vi "motion_ui.vi"() -> ()   [LabVIEW 2012]
uses:
  <vilib>/Platform/TimedLoop/XDataNode/timing_clust.ctl
  <vilib>/Platform/TimedLoop/XDataNode/nitl_modes.ctl
  <vilib>/Platform/TimedLoop/XDataNode/wakeup.ctl
  <vilib>/Platform/TimedLoop/XDataNode/XDataNode.xnode
  <vilib>/Platform/TimedLoop/XDataNode/XDNodeRunTimeDep.lvlib
panel:
  in  "Axis offsets":dbl[](array[numeric])
  in  "Home position":dbl[](array[numeric])
  in  "End transform":dbl[](array[numeric])
  out "Pose":dbl[](array[numeric]) format="%#.4f"
  out "Axis positions":dbl[](array[numeric]) format="%#.4f"
  in  "Continuous":bool
  in  "Go button":bool
  in  "Axis positions ctl":dbl[](array[numeric])=[0.0]
  in  "Position mode":enum16{"Absolute axis", "Relative axis", "Pose"}(ring)
  out "Stopped":bool
  in  "Emergency stop":bool
  in  "Axis names":string[](array[string])
  out "Ready":bool
  in  "Loop":bool
  in  "Step time":dbl=1.0
  out "Executing":i32
  in  "Run sequence":bool
  in  "Sequence":dbl[][](array[numeric])
  in  "stop":bool
  # "Move to"
  # "Move sequence"
  # "Status"
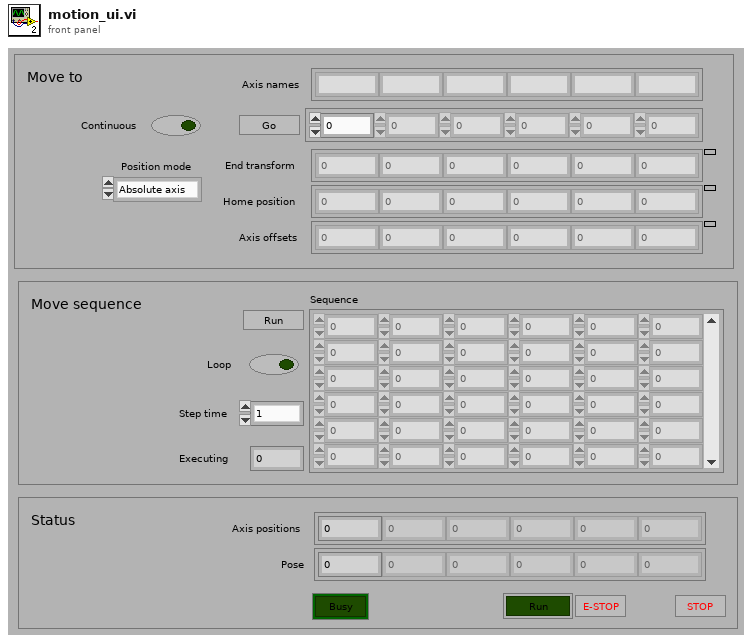
[diagram p1: front panel]
types:
  T1 = typedef "XDNodeRunTimeDep.lvlib/timing_clust.ctl" = cluster{"Expected End [f-1]":u64, "Actual End [f-1]":u64, "Finished Late? [f-1]":bool, "Expected End [i-1]":u64, "Actual End [i-1]":u64, "Finished Late? [i-1]":bool, "Expected Start [i]":u64, "Actual Start [i]":u64, "Expected Start [f]":u64, "Actual Start [f]":u64, "Source Name":string, "Structure Name":string, "Period":i64, "Deadline":i64, "Offset":i64, "Start":i64, "Priority":i32, "Timeout":i32, "Mode":T2, "Wakeup Reason":T3, "Error":errorcluster, "Source Type":string, "Secondary Source Type":string, "Global End Time":u64, "Global Start Time":u64, "Frame Duration":u64, "Iteration Duration":u64, "Assigned CPU":i32, "I/O Scan Engine Mode":u32}
  T2 = typedef "XDNodeRunTimeDep.lvlib/nitl_modes.ctl" = enum32{"No Change", "Process missed periods, maintain original phase", "Discard missed periods, maintain original phase", "Process missed periods, ignore original phase", "Discard missed periods, ignore original phase"}
  T3 = typedef "XDNodeRunTimeDep.lvlib/wakeup.ctl" = enum32{"Normal", "Aborted", "Asynchronous wakeup", "Timing source error", "Timed loop error", "Timeout"}
  T4 = typedef "motion_status.ctl" = cluster{"Axis names":string[], "Axis positions":dbl[], "Pose":dbl[], "Timestamp":u32, "Ready":bool, "Stopped":bool}
  T5 = cluster{"Position mode":enum16{"Absolute axis", "Relative axis", "Pose"}, "Axis positions ctl":dbl[]}
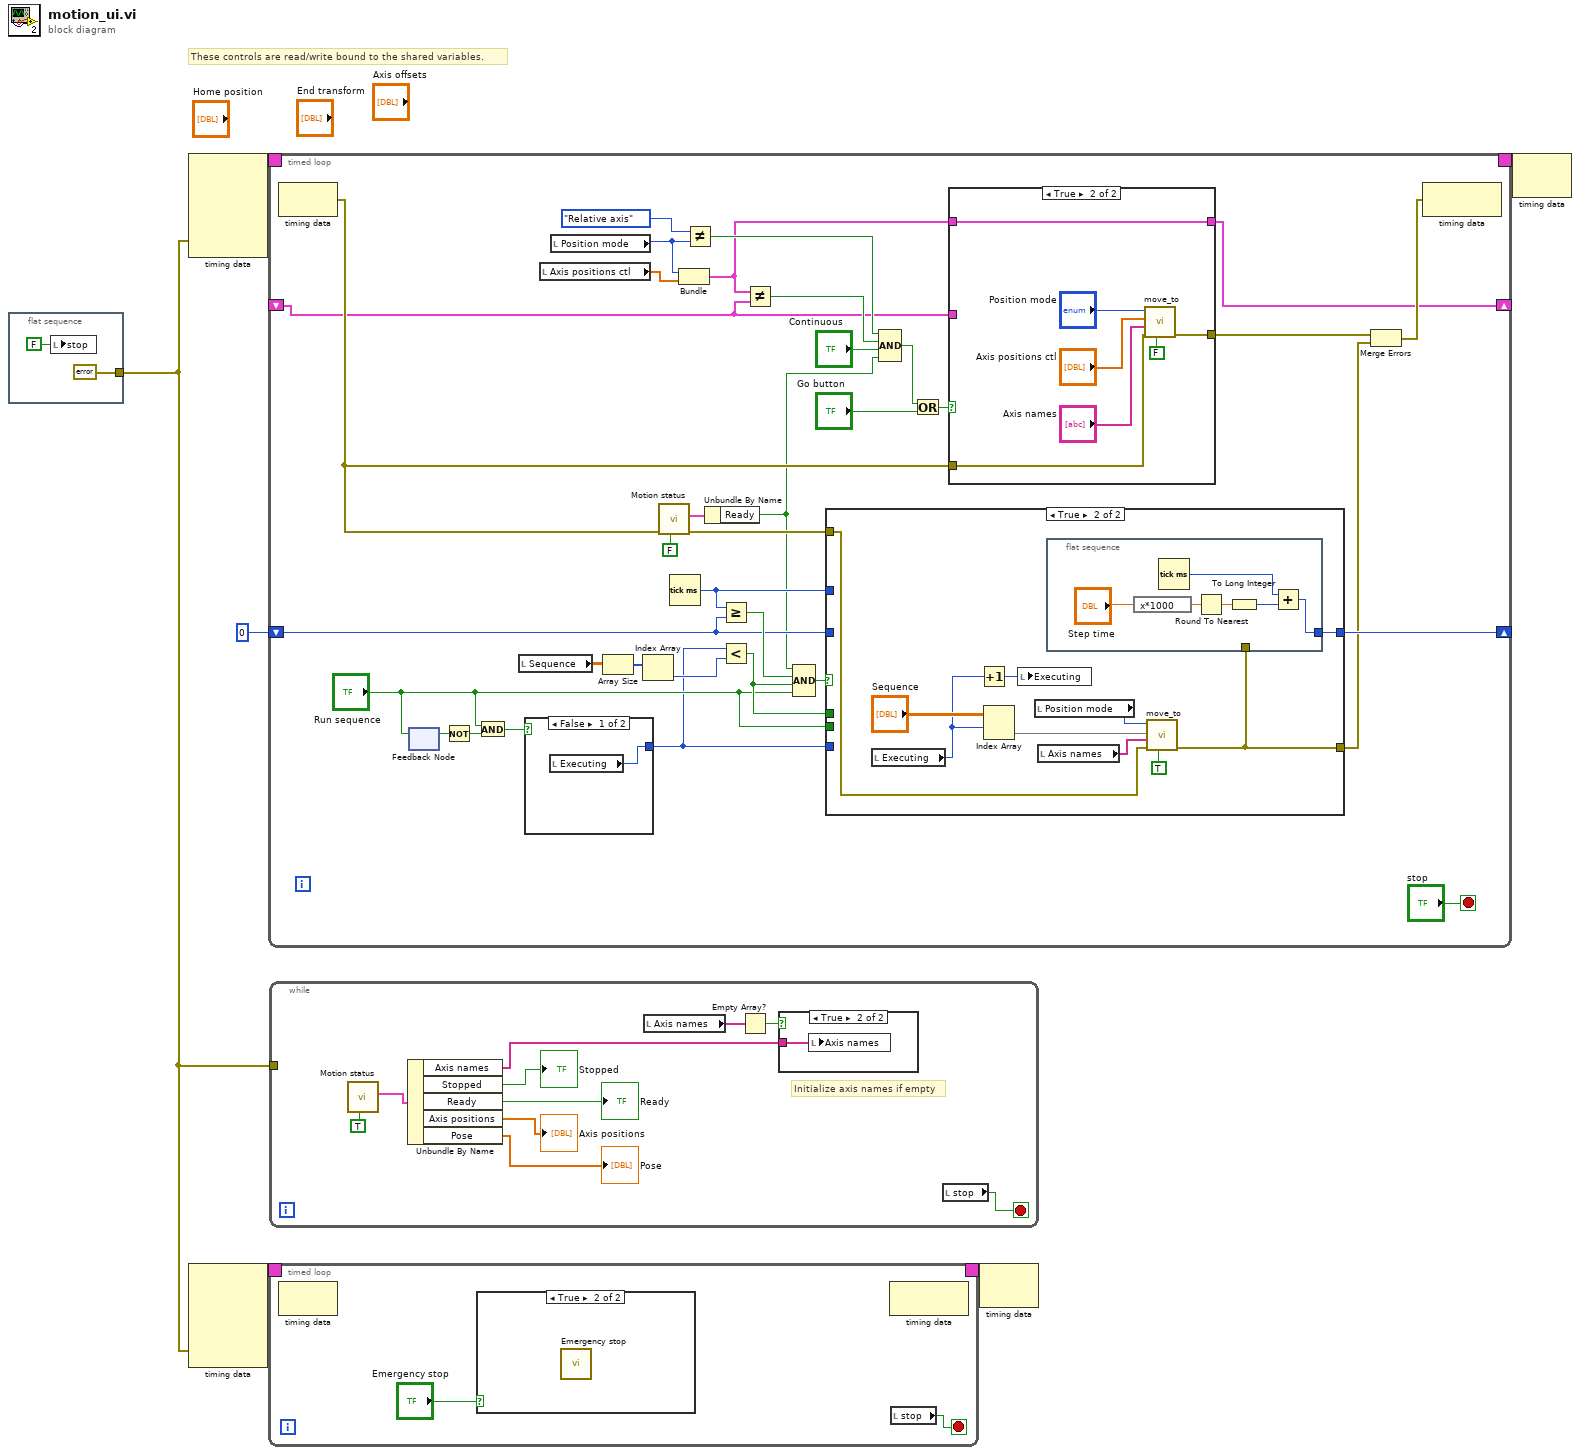
[diagram p0: block diagram]
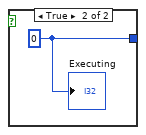
[diagram p4: hidden frame]
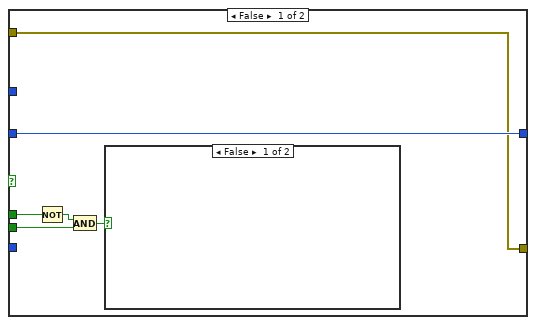
[diagram p5: hidden frame]
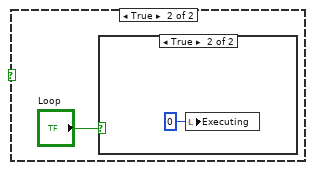
[diagram p6: hidden frame]
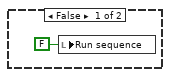
[diagram p7: hidden frame]
diagram:
  # "These controls are read/write bound to the shared variables."
  n1 = flat-sequence {
    tunnel: [errorcluster {"status"=FALSE, "code"=0, "source"=""} ("error out")] -> w1
    frame #0 {
      n2 = local write "stop"(FALSE ("stop")) -> ()
    }
  }
  n3 = node-c288(w1) -> (w6:T1)  [unwired: 4 in]
  n4 = node-c288(w1) -> (w3:T1)  [unwired: 4 in]
  n5 = timed-loop {
    timing: w6 -> [_]
    timing-out: [_] -> w5
    shift-right: [w39] -> _
    shift-left: u32 0 ("millisecond timer value") -> [w29]
    shift-right: [w11] -> _
    shift-left: _ -> [w12]
    stop <- "stop" stop-if-true
    n6 = node-c288() -> (w16:errorcluster)  [unwired: 1 in]
    n7 = feedback-in #1("Run sequence") -> ()
    n8 = feedback #1() -> (w38:bool)  [unwired: 1 in]
    n9 = Not(x=w38) -> (.not. x?=w37:bool)
    n10 = And(x="Run sequence", y=w37) -> (x .and. y?=w36:bool)
    n11 = local read "Sequence"() -> (w35:dbl[][])
    n12 = case shown="False" w36 {
      tunnel: [w44 w45] -> w30
      frame False {
        n13 = local read "Executing"() -> (w44:i32)
      }
      frame True {
        w45 = 0 ("Executing")
        "Executing" <- w45
      }
    }
    n14 = local read "Axis positions ctl"() -> (w25:dbl[])
    n15 = local read "Position mode"() -> (w17:enum16{"Absolute axis", "Relative axis", "Pose"})
    n16 = Array Size(array=w35) -> (size(s)=w34:i32[])
    n17 = Index Array(array=w34) -> (element=w33:i32)  [unwired: 1 in]
    n18 = call "Motion status.vi"("Wait for updated value (F)"=FALSE ("Wait for updated value (T)"), "error in"=w16) -> ("error out"=w26:errorcluster, "Motion status"=w28:T4)  [unwired: 4 in, 4 out]
    n19 = Tick Count (ms)() -> (millisecond timer value=w40:u32)
    n20 = Bundle("Position mode"=w17, "Axis positions ctl"=w25) -> (w10:T5)  [unwired: 1 in]
    n21 = Not Equal?(x=enum16{"Absolute axis", "Relative axis", "Pose"}."Relative axis", y=w17) -> (x != y?=w18:bool)
    n22 = Unbundle By Name(w28) -> ("Ready"=w9:bool)
    n23 = Greater Or Equal?(x=w40, y=w29) -> (x >= y?=w41:bool)
    n24 = Less?(x=w30, y=w33) -> (x < y?=w32:bool)
    n25 = Not Equal?(x=w10, y=w12) -> (x != y?=w24:bool)
    n26 = Compound Arithmetic op=AND(w9, w41, w32, "Run sequence") -> (w42:bool)
    n27 = case shown="True" w42 {
      tunnel: w40 -> [_ _]
      tunnel: [w47 w64] -> w39
      tunnel: w30 -> [_ _]
      tunnel: w32 -> [w51 _]
      tunnel: "Run sequence" -> [w49 _]
      tunnel: w29 -> [w47 _]
      tunnel: w26 -> [w46 w56]
      tunnel: [w46 w55] -> w14
      frame False {
        n28 = Not(x=w51) -> (.not. x?=w50:bool)
        n29 = And(x=w50, y=w49) -> (x .and. y?=w48:bool)
        n30 = case shown="False" w48 {
          frame False {
          }
          frame True {
            n31 = case shown="True" "Loop" {
              frame False {
                n32 = local write "Run sequence"(FALSE ("Run sequence")) -> ()
              }
              frame True {
                n33 = local write "Executing"(0 ("Executing")) -> ()
              }
            }
          }
        }
      }
      frame True {
        n34 = local read "Executing"() -> (w62:i32)
        n35 = Increment(x=w62) -> (x+1=w61:i32)
        n36 = Index Array(array="Sequence", index (row)=w62) -> (element=w59:dbl[])  [unwired: 1 in]
        n37 = local write "Executing"(w61) -> ()
        n38 = local read "Position mode"() -> (w58:enum16{"Absolute axis", "Relative axis", "Pose"})
        n39 = local read "Axis names"() -> (w57:string[])
        n40 = flat-sequence {
          tunnel: [w70] -> w64
          tunnel: w55 -> [_]
          frame #0 {
            n41 = expression code="x*1000"("Step time") -> (w68:dbl)
            n42 = Tick Count (ms)() -> (millisecond timer value=w65:u32)
            n43 = Round To Nearest(number=w68) -> (nearest integer value=w67:dbl)
            n44 = To Long Integer(number=w67) -> (32bit integer=w66:i32)
            n45 = Add(x=w65, y=w66) -> (x+y=w70:u32)
          }
        }
        n46 = call "move_to.vi"("Wait until done"=TRUE, "Error in"=w56, "Axis names"=w57, "Axis positions"=w59, "Mode"=w58) -> ("Error out"=w55:errorcluster)  [unwired: 6 in]
      }
    }
    n47 = Compound Arithmetic op=AND(w18, w24, "Continuous", w9) -> (w20:bool)
    n48 = Or(x=w20, y="Go button") -> (x .or. y?=w21:bool)
    n49 = case shown="True" w21 {
      tunnel: w16 -> [w72 w75]
      tunnel: [w72 w74] -> w13
      tunnel: [w71 w73] -> w11
      tunnel: w12 -> [w71 _]
      tunnel: w10 -> [_ w73]
      frame False {
      }
      frame True {
        n50 = call "move_to.vi"("Wait until done"=FALSE, "Error in"=w75, "Axis names"="Axis names", "Axis positions"="Axis positions ctl", "Mode"="Position mode") -> ("Error out"=w74:errorcluster)  [unwired: 6 in]
      }
    }
    n51 = Merge Errors(w13, w14) -> (w15:errorcluster)
    n52 = node-c288(w15) -> ()  [unwired: 1 out]
  }
  n53 = timed-loop {
    timing: w3 -> [_]
    timing-out: [_] -> w2
    stop <- w85 stop-if-true
    n54 = node-c288() -> ()  [unwired: 1 in, 1 out]
    n55 = case shown="True" "Emergency stop" {
      frame False {
      }
      frame True {
        n56 = call "Emergency stop.vi"() -> ()  [unwired: 11 in, 1 out]
      }
    }
    n57 = node-c288() -> ()  [unwired: 1 in, 1 out]
    n58 = local read "stop"() -> (w85:bool)
  }
  n59 = while {
    tunnel: w1 -> [_]
    stop <- w98 stop-if-true
    # "Initialize axis names if empty"
    n60 = call "Motion status.vi"("Wait for updated value (F)"=TRUE) -> ("Motion status"=w97:T4)  [unwired: 5 in, 5 out]
    n61 = Unbundle By Name(w97) -> ("Axis names"=w90:string[], "Stopped"=→"Stopped":bool, "Ready"=→"Ready":bool, "Axis positions"=→"Axis positions":dbl[], "Pose"=→"Pose":dbl[])
    n62 = local read "Axis names"() -> (w92:string[])
    n63 = Empty Array?(array=w92) -> (empty?=w91:bool)
    n64 = case shown="True" w91 {
      tunnel: w90 -> [_ w99]
      frame False {
      }
      frame True {
        n65 = local write "Axis names"(w99) -> ()
      }
    }
    n66 = local read "stop"() -> (w98:bool)
  }
  n67 = node-c288(w2) -> ()  [unwired: 1 out]
  n68 = node-c288(w5) -> ()  [unwired: 1 out]
